vi "select_data_timezone.vi"(7 "connection_reference":T1, 8 "error in (no error)":errorcluster, 9 "timezone":string="UTC", 10 "range_finish":dbl format="%^<%H:%M:%S%4u %m/%d/%y>T", 11 "range_start":dbl format="%^<%H:%M:%S%4u %m/%d/%y>T") -> (0 "error out":errorcluster, 3 "data_read":cluster{"time":dbl, "value":dbl}[](array[cluster]) {"value" format="%#_10f"; "time" format="%^<%H:%M:%S%3u %m/%d/%y>T"})   [LabVIEW 2015, in "lv-example-postgres.lvlib"]
uses:
  lv-example-postgres.lvlib
  <vilib>/addons/database/Connection.llb/Conn ObjectReference.ctl
  <vilib>/addons/database/Command.llb/Cmd Execute.vi
  <vilib>/addons/database/Recordset.llb/Rec Fetch Recordset Data (CR).vi
  <vilib>/addons/database/Recordset.llb/Rec Destroy - Command.vi
  <vilib>/addons/database/Command.llb/Cmd Delete.vi
  <vilib>/addons/database/NI_Database_API.lvlib
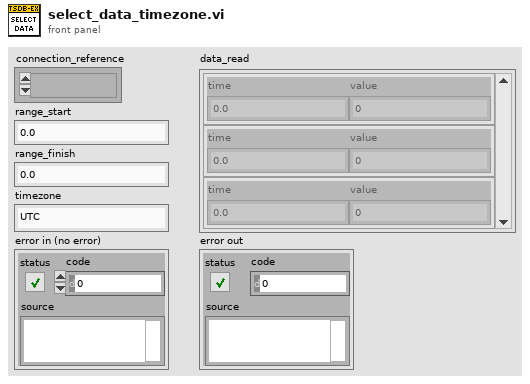
[diagram p1: front panel]
types:
  T1 = typedef "NI_Database_API.lvlib/Conn ObjectReference.ctl" = refnum<k1>
  T2 = cluster{"timezone":string, "postgres_date":string}
  T3 = typedef "NI_Database_API.lvlib/DB Tools Parameter Info.ctl" = cluster{"parameter name":string, "type":T4, "direction":T5, "value":variant}
  T4 = typedef "NI_Database_API.lvlib/DB Tools DataTypes.ctl" = enum16{"String", "Long (I32)", "Single (SGL)", "Double (DBL)", "Date/Time", "Binary"}
  T5 = typedef "NI_Database_API.lvlib/DB Tools Parameter Dir.ctl" = enum32{"Input", "Output", "Input/Output", "Return Value"}
  T6 = typedef "NI_Database_API.lvlib/Cmd ObjectReference.ctl" = refnum<k1>
  T7 = typedef "NI_Database_API.lvlib/Cmd-Rec Object Reference.ctl" = refnum<k1>
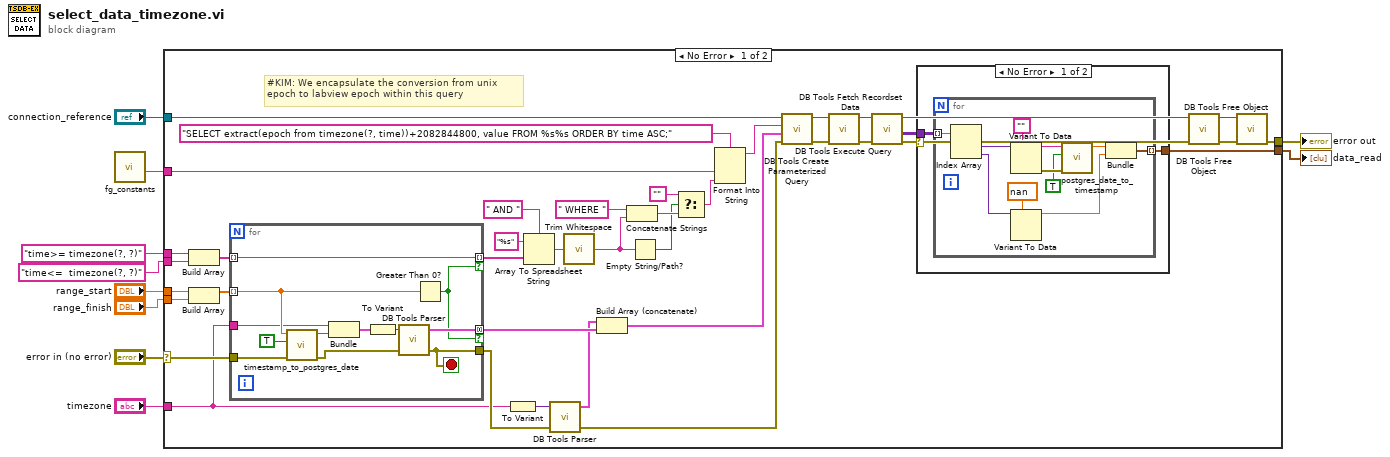
[diagram p0: block diagram]
diagram:
  n1 = call "fg_constants.vi"() -> ("table out"=w1:string)  [unwired: 9 in, 2 out]
  n2 = case shown="No Error" "error in (no error)" {
    selector: "error in (no error)" -> [w42 w75]
    tunnel: [w48 _] -> w4
    tunnel: w1 -> [w21 _]
    tunnel: "connection_reference" -> [w25 _]
    tunnel: [w12 w75] -> w5
    tunnel: "range_start" -> [w44 _]
    tunnel: "range_finish" -> [w43 _]
    tunnel: "time>= timezone(?, ?)" ("format string") -> [w46 _]
    tunnel: "time<=  timezone(?, ?)" ("format string") -> [w45 _]
    tunnel: "timezone" -> [w16 _]
    frame No Error {
      # "#KIM: We encapsulate the conversion from unix\nepoch to labview epoch within this query"
      n3 = Build Array(w46, w45) -> (w23:string[])
      n4 = Build Array(w44, w43) -> (w37:dbl[])
      n5 = for {
        tunnel: w23 -> [w66] mode=indexing
        tunnel: w37 -> [w73] mode=indexing
        tunnel: [w66] -> w35 mode=indexing if=w67
        tunnel: [w68] -> w20 mode=concatenating if=w67
        tunnel: w16 -> [w64]
        tunnel: w42 -> [w74]
        tunnel: [w70] -> w49
        stop <- w70 stop-if-true
        n6 = call "timestamp_to_postgres_date.vi"("error in (no error)"=w74, "utc"=TRUE, "date_time"=w73) -> ("error out"=w71:errorcluster, "postgres_date"=w63:string)  [unwired: 7 in]
        n7 = Bundle("timezone"=w64, "postgres_date"=w63) -> (w65:T2)  [unwired: 1 in]
        n8 = To Variant(anything=w65) -> (Variant=w69:variant)
        n9 = call <vilib>:"DB Tools Parser.vi"("error in (no error)"=w71, "variant"=w69) -> ("error out"=w70:errorcluster, "parameters"=w68:T3[])  [unwired: 2 in]
        n10 = Greater Than 0?(x=w73) -> (x > 0?=w67:bool)
      }
      n11 = To Variant(anything=w16) -> (Variant=w14:variant)
      n12 = Array To Spreadsheet String(delimiter (Tab)=" AND " ("format string"), array=w35, 3:"%s" ("format string")) -> (spreadsheet string=w39:string)
      n13 = call <vilib>:"DB Tools Parser.vi"("error in (no error)"=w49, "variant"=w14) -> ("error out"=w15:errorcluster, "parameters"=w17:T3[])  [unwired: 2 in]
      n14 = call <vilib>:"Trim Whitespace.vi"("string"=w39) -> ("trimmed string"=w33:string)  [unwired: 1 in]
      n15 = Build Array (concatenate)(w17, w20) -> (w18:T3[])
      n16 = Concatenate Strings(" WHERE " ("format string"), w33) -> (w34:string)
      n17 = Empty String/Path?(string/path=w33) -> (empty?=w32:bool)
      n18 = Select(t="", s=w32, f=w34) -> (s? t:f=w22:string)
      n19 = Format Into String(format string="SELECT extract(epoch from timezone(?, time))+2082844800, value FROM %s%s ORDER BY time ASC;", w21, w22) -> (resulting string=w24:string)  [unwired: 2 in, 1 out]
      n20 = call <vilib>:"DB Tools Create Parameterized Query.vi"("error in (no error)"=w15, "parameters"=w18, "SQL query"=w24, "connection reference"=w25) -> ("error out"=w31:errorcluster, "command reference"=w30:T6)  [unwired: 3 in, 1 out]
      n21 = call-poly <vilib>:"DB Tools Execute Query.vi"("error in (no error)"=w31, "command reference"=w30) -> ("error out"=w28:errorcluster, "command-recordset reference"=w27:T7)  [unwired: 6 in]
      n22 = call-poly <vilib>:"DB Tools Fetch Recordset Data.vi"("error in (no error)"=w28, "command-recordset reference"=w27) -> ("error out"=w11:errorcluster, "recordset data"=w19:variant[][], "command-recordset reference out"=w26:T7)  [unwired: 3 in]
      n23 = case shown="No Error" w11 {
        tunnel: [w51 _] -> w48
        tunnel: w19 -> [w50 _]
        frame No Error {
          n24 = for {
            tunnel: w50 -> [w62] mode=indexing
            tunnel: [w52] -> w51 mode=indexing
            n25 = Index Array(array=w62) -> (element #1=w61:variant, element #2=w60:variant)  [unwired: 2 in]
            n26 = Variant To Data(type="", Variant=w61) -> (data=w57:string, error out=w56:errorcluster)  [unwired: 1 in]
            n27 = Variant To Data(type=nan, Variant=w60) -> (data=w53:dbl)  [unwired: 1 in, 1 out]
            n28 = call "postgres_date_to_timestamp.vi"("error in (no error)"=w56, "utc"=TRUE, "postgres_date"=w57) -> ("date_time"=w54:dbl)  [unwired: 7 in, 1 out]
            n29 = Bundle("date_time"=w54, w53) -> (w52:cluster{"date_time":dbl, dbl})  [unwired: 1 in]
          }
        }
        frame Error {
        }
      }
      n30 = call-poly <vilib>:"DB Tools Free Object.vi"("error in (no error)"=w11, "command-recordset reference"=w26) -> ("error out"=w13:errorcluster, "command reference"=w29:T6)  [unwired: 8 in]
      n31 = call-poly <vilib>:"DB Tools Free Object.vi"("error in (no error)"=w13, "command reference"=w29) -> ("error out"=w12:errorcluster)  [unwired: 8 in, 1 out]
    }
    frame Error {
    }
  }
  "data_read" <- w4
  "error out" <- w5
